vi "to variant array.vi"(11 "Variant":variant) -> (3 "Array":variant[](array[variant]))   [LabVIEW 2019]
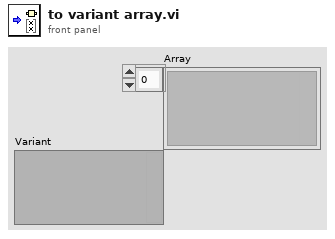
[diagram p1: front panel]
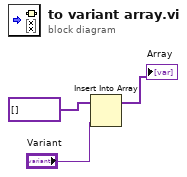
[diagram p0: block diagram]
diagram:
  n1 = Insert Into Array(array=variant[] [], new element="Variant") -> (→"Array":variant[])  [unwired: 1 in]
